vi "transition.vi"(4 "previous_state":T1, 6 "current_state":T1, 7 "transition_queue":refnum<queue>, 8 "error in (no error)":errorcluster, 9 "step":string, 10 "index in":i32, 11 "recipe_data in":variant) -> (0 "error out":errorcluster, 2 "index out":i32, 3 "recipe_data out":variant)   [LabVIEW 2015, in "example_02.lvlib"]
uses:
  example_02.lvlib
  <userlib>/antonio-alexander/lv-recipe-machine/public/_controls/automatic_state.ctl
  <userlib>/antonio-alexander/lv-recipe-machine/public/_controls/transition.ctl
  <userlib>/antonio-alexander/lv-recipe-machine/lv-recipe-machine.lvlib
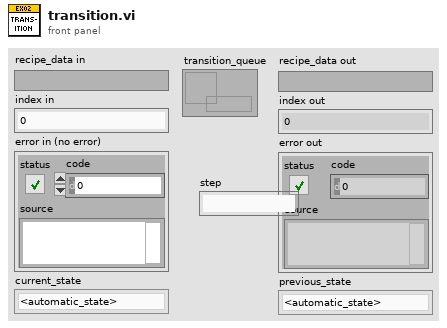
[diagram p1: front panel]
types:
  T1 = typedef "lv-recipe-machine.lvlib/automatic_state.ctl" = enum16{"<automatic_state>", "failed", "idle", "running", "paused", "stopped", "<null>"}
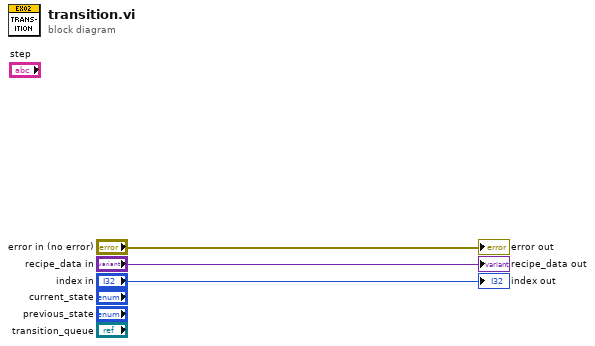
[diagram p0: block diagram]
diagram:
  "error out" <- "error in (no error)"
  "recipe_data out" <- "recipe_data in"
  "index out" <- "index in"
